vi "validate_password.vi"(11 "Password":string) -> (3 "Accept":bool)   [LabVIEW 2013, in "main.lvlib"]
uses:
  main.lvlib
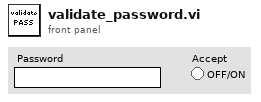
[diagram p1: front panel]
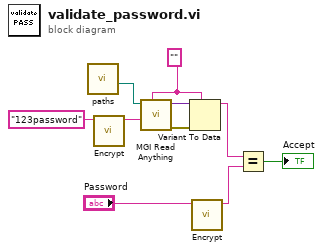
[diagram p0: block diagram]
diagram:
  w3 = ""
  n1 = call "paths.vi"() -> ("Controlsettings2"=w4:path)  [unwired: 8 in, 3 out]
  n2 = call "Encrypt.vi"("Input"="123password") -> ("Output"=w5:string)  [unwired: 10 in]
  n3 = call <userlib>:"MGI Read Anything.vi"("Type of Anything"=w3, "Section Name (Name of \"Type of Anything\")"=w5, "Path (dialog)"=w4) -> ("Error Out"=w1:errorcluster, "Anything"=w2:variant)  [unwired: 5 in, 2 out]
  n4 = Variant To Data(error in=w1, type=w3, Variant=w2) -> (data=w9:string)  [unwired: 1 out]
  n5 = call "Encrypt.vi"("Input"="Password") -> ("Output"=w8:string)  [unwired: 10 in]
  n6 = Equal?(x=w9, y=w8) -> (x = y?=→"Accept":bool)
